vi "init_3D Model.vi"(8 "error in":errorcluster) -> (0 "error out":errorcluster, 1 "Scene Object Out":refnum<vi>, 3 "myRIO ref":refnum<vi>)   [LabVIEW 2019]
doc: "This VI initialize the 3D Viewer part which reads myRIO CAD Model and generates Geodetic Coordinate System. Then it adjusts the size of both myRIO and the Coordinate System."
uses:
  <vilib>/picture/3D Picture Control/NI_3D Picture Control.lvlib
  <vilib>/picture/3D Picture Control/Object/Add Object (no reference).vi
  <vilib>/picture/3D Picture Control/Object/Create Object (name).vi
panel:
  # "This VI initialize the 3D Viewer part which reads myRIO CAD\nModel and generates Geodetic Coordinate System. Then it ajdusts \nthe size of both myRIO and the Coordinate System."
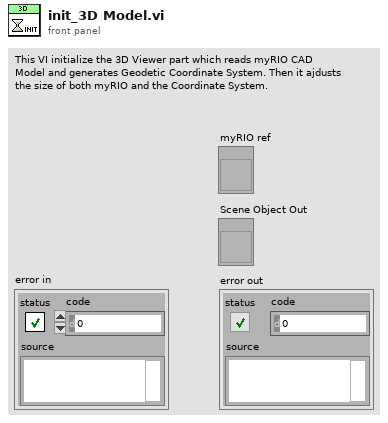
[diagram p1: front panel]
types:
  T1 = cluster{"Red":sgl, "Green":sgl, "Blue":sgl, "Alpha":sgl}
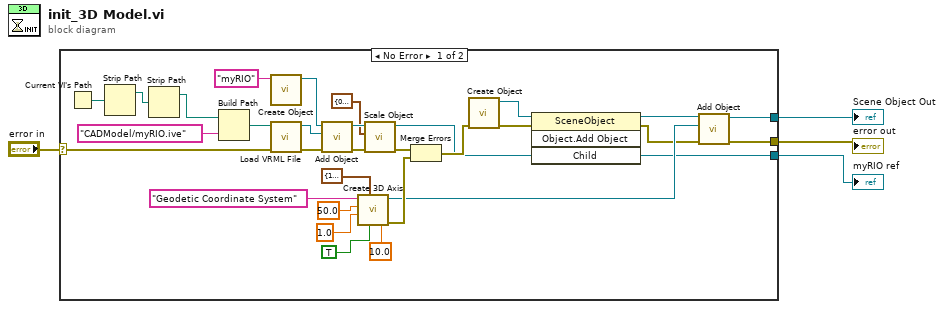
[diagram p0: block diagram]
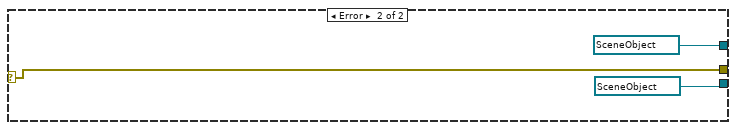
[diagram p2: hidden frame]
diagram:
  n1 = case shown="No Error" "error in" {
    selector: "error in" -> [w19 w38]
    tunnel: [w15 w38] -> w2
    tunnel: [w14 refnum<vi> refnum ("Scene Object Out")] -> w3
    tunnel: [w6 refnum<vi> refnum ("Child")] -> w1
    frame No Error {
      n2 = Current VI's Path() -> (path=w31:path)
      n3 = Strip Path(path=w31) -> (stripped path=w13:path)  [unwired: 1 out]
      n4 = Strip Path(path=w13) -> (stripped path=w12:path)  [unwired: 1 out]
      n5 = Build Path(base path=w12, name or relative path="CADModel/myRIO.ive") -> (appended path=w29:path)
      n6 = call-poly <vilib>:"Create Object.vi"("Name"="myRIO") -> ("Scene:New Object"=w28:refnum<vi>)  [unwired: 9 in, 1 out]
      n7 = call <vilib>:"Load VRML File.vi"("error in"=w19, "Path"=w29) -> ("error out"=w25:errorcluster, "Scene:Read Scene File"=w26:refnum<vi>)  [unwired: 8 in]
      n8 = call-poly <vilib>:"Add Object.vi"("error in (no error)"=w25, "New Object In"=w26, "Scene Object In"=w28) -> ("error out"=w23:errorcluster, "Scene Object Out"=w24:refnum<vi>)  [unwired: 7 in]
      n9 = call <vilib>:"Create 3D Axis.vi"("Character Size"=sgl 10.0, "Axis label?"=TRUE, "Color"=T1 {"Red"=1.0, "Green"=1.0, "Blue"=1.0, "Alpha"=1.0}, "Radius"=sgl 1.0, "Length"=sgl 50.0, "Name"="Geodetic Coordinate System") -> ("error out"=w17:errorcluster, "New Object Refnum"=w8:refnum<vi>)  [unwired: 4 in]
      n10 = call <vilib>:"Scale Object.vi"("error in (no error)"=w23, "Scale"=cluster{"X":sgl, "Y":sgl, "Z":sgl} {"X"=0.3, "Y"=0.3, "Z"=0.3}, "Scene.Object In"=w24) -> ("error out"=w18:errorcluster, "Scene.Object Out"=w9:refnum<vi>)  [unwired: 7 in]
      n11 = Merge Errors(w18, w17) -> (w16:errorcluster)
      n12 = call-poly <vilib>:"Create Object.vi"("error in (no error)"=w16) -> ("error out"=w10:errorcluster, "Scene:New Object"=w11:refnum<vi>)  [unwired: 9 in]
      n13 = invoke class="SceneObject" method="Object.Add Object"(reference=w11, error in=w10, "Child"=w9) -> (reference out=w7:refnum<vi>, error out=w5:errorcluster, "Child"=w6:refnum<vi>)  [unwired: 1 in, 1 out]
      n14 = call-poly <vilib>:"Add Object.vi"("error in (no error)"=w5, "New Object In"=w8, "Scene Object In"=w7) -> ("error out"=w15:errorcluster, "Scene Object Out"=w14:refnum<vi>)  [unwired: 7 in]
    }
    frame Error {
    }
  }
  "Scene Object Out" <- w3
  "error out" <- w2
  "myRIO ref" <- w1
